vi "scantimingsource_10ms_1dt.vi"() -> (0 "max jitter (uS)":dbl format="%.2f", 1 "mean time (uS)":dbl format="%.2f", 2 "standard deviation (uS)":dbl format="%.2f", 3 "execution histogram":T1(graph), 4 "Error":errorcluster, 5 "execution times (uS)":dbl[](graph))   [LabVIEW 2013]
uses:
  <vilib>/Platform/TimedLoop/XDataNode/timing_clust.ctl
  <vilib>/Platform/TimedLoop/XDataNode/nitl_modes.ctl
  <vilib>/Platform/TimedLoop/XDataNode/wakeup.ctl
  <vilib>/Platform/TimedLoop/XDataNode/loadnilvce.vi
  <vilib>/platform/TimedLoop/XDataNode/XDataNode.xnode
  <vilib>/Platform/TimedLoop/XDataNode/XDNodeRunTimeDep.lvlib
  <vilib>/NI_Real-Time Target Support.lvlib
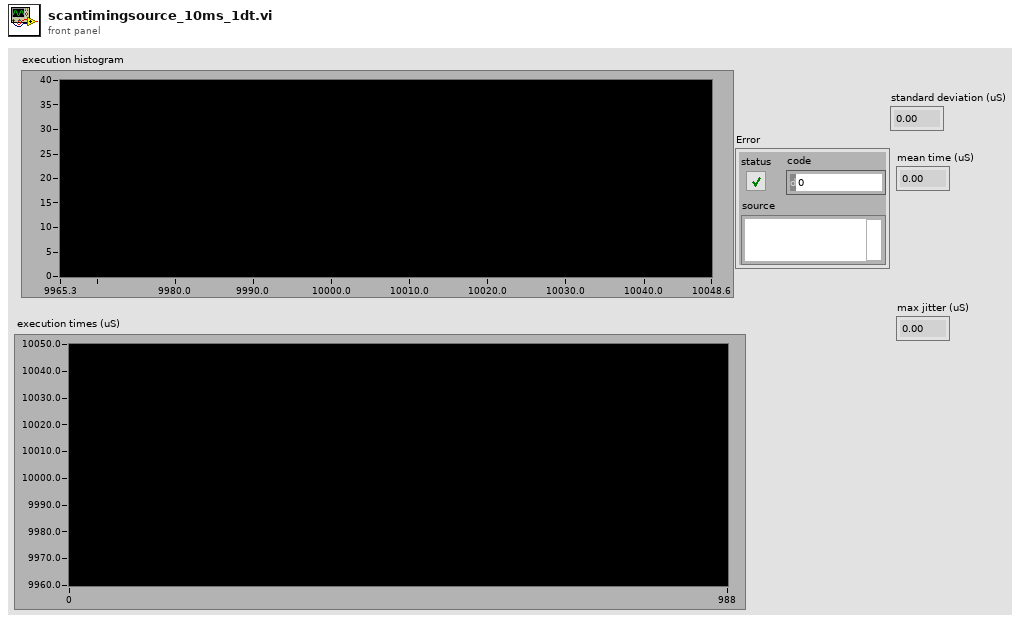
[diagram p1: front panel]
types:
  T1 = cluster{"X Values":dbl[], "Histogram: h(x)":i32[]}
  T2 = typedef "XDNodeRunTimeDep.lvlib/timing_clust.ctl" = cluster{"Expected End [f-1]":u64, "Actual End [f-1]":u64, "Finished Late? [f-1]":bool, "Expected End [i-1]":u64, "Actual End [i-1]":u64, "Finished Late? [i-1]":bool, "Expected Start [i]":u64, "Actual Start [i]":u64, "Expected Start [f]":u64, "Actual Start [f]":u64, "Source Name":string, "Structure Name":string, "Period":i64, "Deadline":i64, "Offset":i64, "Start":i64, "Priority":i32, "Timeout":i32, "Mode":T3, "Wakeup Reason":T4, "Error":errorcluster, "Source Type":string, "Secondary Source Type":string, "Global End Time":u64, "Global Start Time":u64, "Frame Duration":u64, "Iteration Duration":u64, "Assigned CPU":i32, "I/O Scan Engine Mode":u32}
  T3 = typedef "XDNodeRunTimeDep.lvlib/nitl_modes.ctl" = enum32{"No Change", "Process missed periods, maintain original phase", "Discard missed periods, maintain original phase", "Process missed periods, ignore original phase", "Discard missed periods, ignore original phase"}
  T4 = typedef "XDNodeRunTimeDep.lvlib/wakeup.ctl" = enum32{"Normal", "Aborted", "Asynchronous wakeup", "Timing source error", "Timed loop error", "Timeout"}
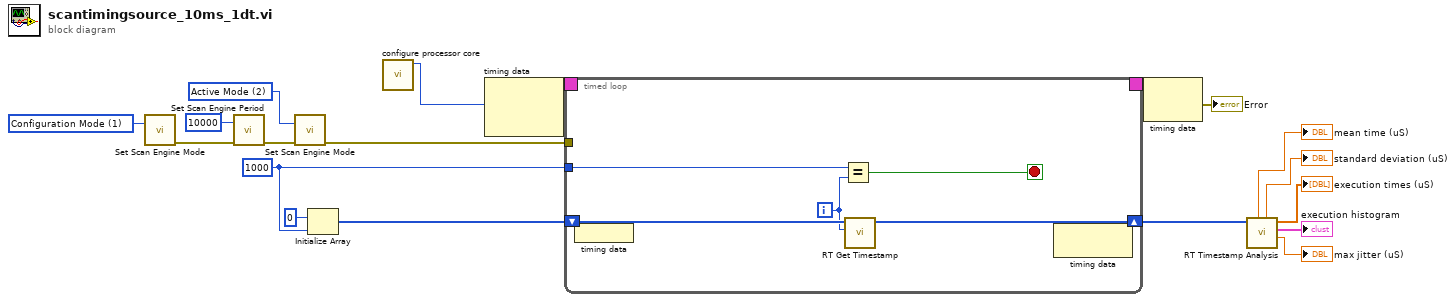
[diagram p0: block diagram]
diagram:
  w11 = 1000 ("x")
  w16 = 1 items=["Configuration Mode"=1, "Active Mode"=2] ("mode (Active Mode)")
  w17 = 2 items=["Configuration Mode"=1, "Active Mode"=2] ("mode (Active Mode)")
  n1 = call <vilib>:"Set Scan Engine Mode.vi"("mode (Active Mode)"=w16) -> ("error out"=w18:errorcluster)  [unwired: 14 in]
  n2 = call <vilib>:"Set Scan Engine Period.vi"("scan period (uSec)"=u32 10000, "error in (no error)"=w18) -> ("error out"=w19:errorcluster)  [unwired: 13 in]
  n3 = call <vilib>:"Set Scan Engine Mode.vi"("mode (Active Mode)"=w17, "error in (no error)"=w19) -> ("error out"=w14:errorcluster)  [unwired: 13 in]
  n4 = Initialize Array(u64 0, w11) -> (w12:u64[])
  n5 = call "configure processor core.vi"() -> ("Processor"=w1:i32)  [unwired: 11 in]
  n6 = node-c288(w1) -> (w4:T2)  [unwired: 1 in]
  n7 = timed-loop {
    timing: w4 -> [_]
    timing-out: [_] -> w3
    tunnel: w14 -> [_]
    shift-right: [w21] -> w10
    shift-left: w12 -> [w22]
    tunnel: w11 -> [w24]
    i -> [w20]
    stop <- w23 stop-if-true
    n8 = node-c288() -> ()  [unwired: 1 in]
    n9 = Equal?(x=w24, y=w20) -> (x = y?=w23:bool)
    n10 = call <vilib>:"RT Get Timestamp.vi"("iteration"=w20, "timestamp array in"=w22) -> ("timestamp array out"=w21:u64[])  [unwired: 8 in, 1 out]
    n11 = node-c288() -> ()  [unwired: 1 in, 1 out]
  }
  n12 = node-c288(w3) -> (→"Error":errorcluster)
  n13 = call <vilib>:"RT Timestamp Analysis.vi"("timestamp array"=w10) -> ("max jitter (uS)"=→"max jitter (uS)":dbl, "execution histogram"=→"execution histogram":T1, "execution times (uS)"=→"execution times (uS)":dbl[], "standard deviation (uS)"=→"standard deviation (uS)":dbl, "mean time (uS)"=→"mean time (uS)":dbl)  [unwired: 5 in, 1 out]
